vi "X Axis Motor Speed Controller (1).vi"(1 "Speed Command (mm/s)":dbl) -> (0 "PWM  Duty Cycle Command (Hz)":dbl)   [LabVIEW 2013]
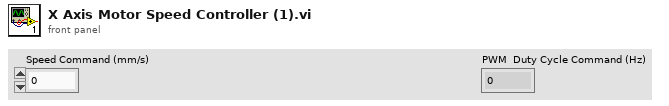
[diagram p1: front panel]
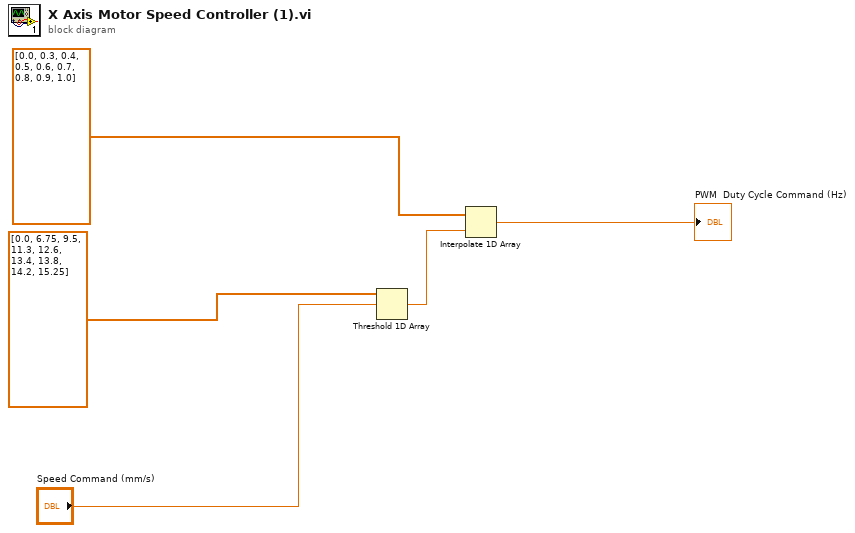
[diagram p0: block diagram]
diagram:
  n1 = Threshold 1D Array(2:"Speed Command (mm/s)", 3:dbl[] [0.0, 6.75, 9.5, 11.3, 12.6, 13.4, 13.8, 14.2, 15.25] ("Speed")) -> (0:w3:dbl)  [unwired: 1 in]
  n2 = Interpolate 1D Array(1:w3, 2:dbl[] [0.0, 0.3, 0.4, 0.5, 0.6, 0.7, 0.8, 0.9, 1.0] ("Duty Cycle")) -> (0:→"PWM  Duty Cycle Command (Hz)":dbl)
